vi "Migrate Dependencies.vi"(0 "Project path":path, 5 "Measurement paths":path[](array[path]), 7 "Plug-in names":string[](array[string]), 9 "Progress":refnum<vi>, 11 "error in":errorcluster) -> (4 "Instrument containing subVIs":path[][](array[path]), 15 "error out":errorcluster)   [LabVIEW 2021, in "Multiple Converter.lvlib"]
doc: "Convert multiple measurements along with their dependencies, either dependencies being shared among measurements or measurements having their own depenencies."
uses:
  Multiple Converter.lvlib
panel:
  # "Dependencies Migration"
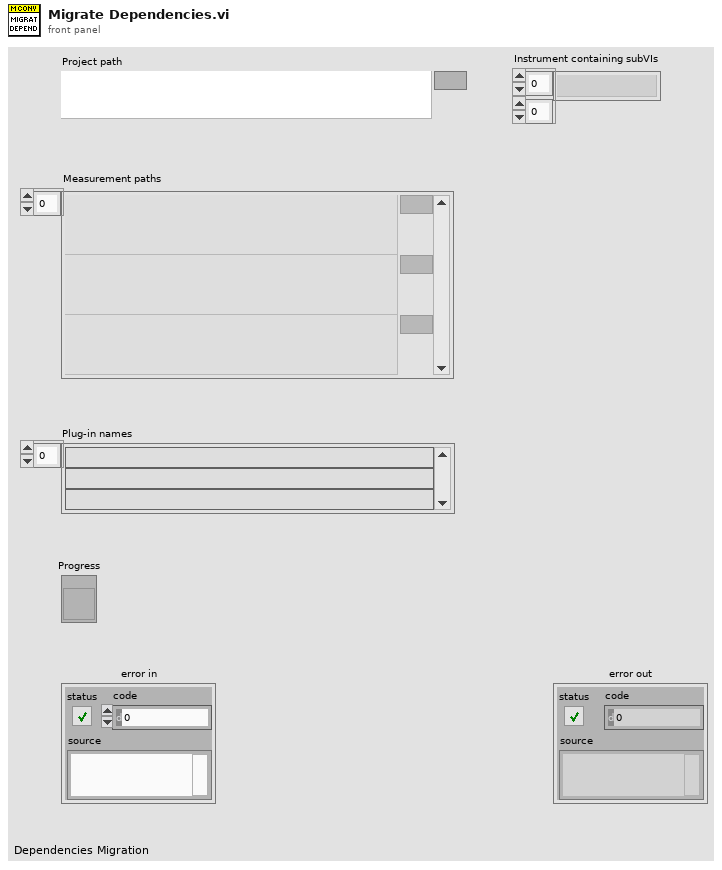
[diagram p1: front panel]
types:
  T1 = typedef "Multiple Converter.lvlib/Library Info.ctl" = cluster{"Library path":path, "Library name":string}
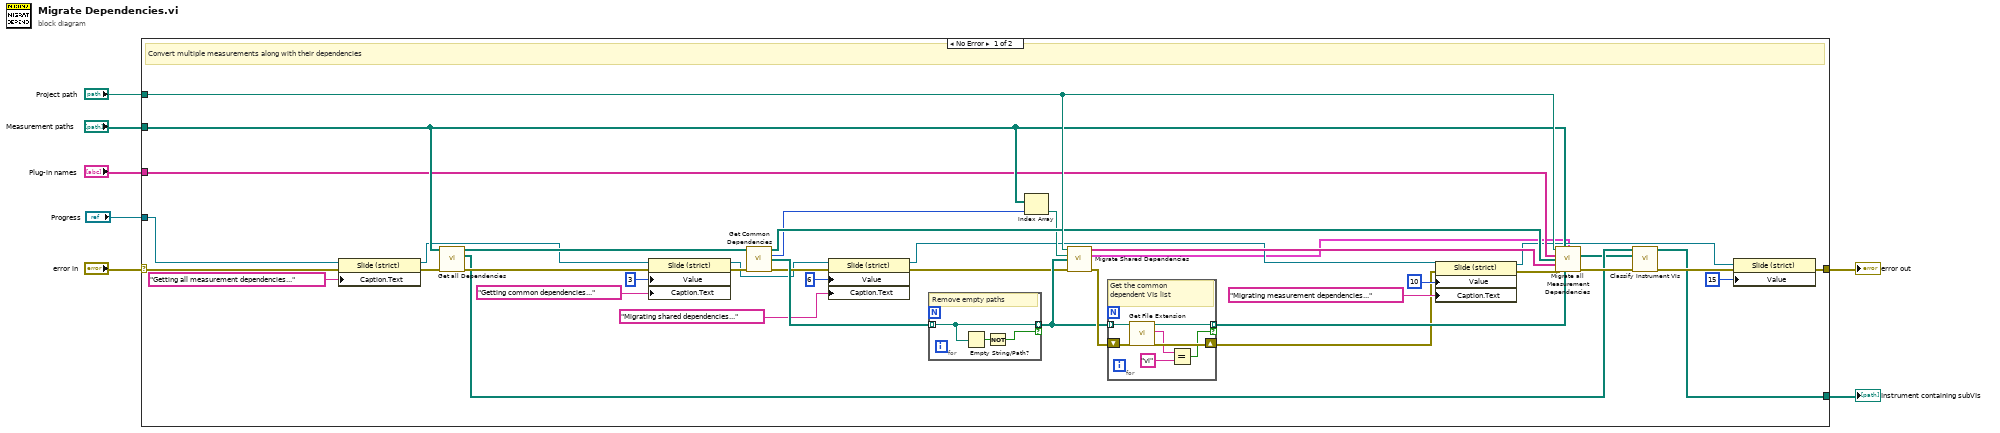
[diagram p0: block diagram]
diagram:
  n1 = case shown="No Error" "error in" {
    selector: "error in" -> [w35 w58]
    tunnel: "Project path" -> [w47 _]
    tunnel: "Measurement paths" -> [w46 _]
    tunnel: "Plug-in names" -> [w45 _]
    tunnel: [w16 w58] -> w4
    tunnel: [w10 _] -> w2
    tunnel: "Progress" -> [w33 _]
    frame No Error {
      # "Convert multiple measurements along with their dependencies"
      n2 = property class="Slide (strict)"(reference=w33, error in=w35, "Caption.Text"="Getting all measurement dependencies...") -> (reference out=w28:refnum<vi>, error out=w34:errorcluster)
      n3 = call "Get all Dependencies.vi"("Measurement paths"=w46, "error in (no error)"=w34) -> ("All dependencies"=w44:path[][], "Instrument containing subVIs"=w11:path[][], "error out"=w31:errorcluster)  [unwired: 11 in]
      n4 = property class="Slide (strict)"(reference=w28, error in=w31, "Value"=3, "Caption.Text"="Getting common dependencies...") -> (reference out=w22:refnum<vi>, error out=w30:errorcluster)
      n5 = call "Get Common Dependencies.vi"("All dependencies"=w44, "error in (no error)"=w30) -> ("Measurement dependencies"=w43:path[][], "Measurement index"=w37:i32, "Common dependencies"=w38:path[], "error out"=w24:errorcluster)  [unwired: 10 in]
      n6 = property class="Slide (strict)"(reference=w22, error in=w24, "Value"=6, "Caption.Text"="Migrating shared dependencies...") -> (reference out=w15:refnum<vi>, error out=w23:errorcluster)
      n7 = for {
        tunnel: [w48] -> w36 mode=indexing if=w49
        tunnel: w38 -> [w48] mode=indexing
        # "Remove empty paths"
        n8 = Empty String/Path?(string/path=w48) -> (empty?=w50:bool)
        n9 = Not(x=w50) -> (.not. x?=w49:bool)
      }
      n10 = Index Array(array=w46, index=w37) -> (element=w39:path)
      n11 = call "Migrate Shared Dependencies.vi"("Project path"=w47, "Measurement path"=w39, "Common dependencies"=w36, "error in (no error)"=w23) -> ("Outside items"=w42:string[], "Library"=w8:T1[], "error out"=w40:errorcluster)  [unwired: 9 in]
      n12 = for {
        shift-right: [w56] -> w19
        shift-left: w40 -> [w57]
        tunnel: [w52] -> w41 mode=indexing if=w53
        tunnel: w36 -> [w51] mode=indexing
        # "Get the common dependent VIs list"
        n13 = call <vilib>:"Get File Extension.vi"("error in (no error)"=w57, "file"=w51) -> ("error out"=w56:errorcluster, "lowercase file extension"=w54:string, "dup file"=w52:path)  [unwired: 5 in, 2 out]
        n14 = Equal?(x=w54, y="vi" ("x")) -> (x = y?=w53:bool)
      }
      n15 = property class="Slide (strict)"(reference=w15, error in=w19, "Value"=10, "Caption.Text"="Migrating measurement dependencies...") -> (reference out=w14:refnum<vi>, error out=w18:errorcluster)
      n16 = call "Migrate all Measurement Dependencies.vi"("Project path"=w47, "Measurement paths"=w46, "Init"=w8, "Plug-in names"=w45, "Measurement dependencies"=w43, "Outside items"=w42, "error in (no error)"=w18, "Shared dependent VIs"=w41) -> ("DestinationDirectory"=w9:path[], "error out"=w13:errorcluster)  [unwired: 6 in]
      n17 = call "Classify Instrument VIs.vi"("InstrContaining"=w11, "DestinationDirectory"=w9, "error in (no error)"=w13) -> ("InstrContainingVI[]"=w10:path[][], "error out"=w12:errorcluster)  [unwired: 11 in]
      n18 = property class="Slide (strict)"(reference=w14, error in=w12, "Value"=15) -> (error out=w16:errorcluster)  [unwired: 1 out]
    }
    frame Error {
    }
  }
  "error out" <- w4
  "Instrument containing subVIs" <- w2
